vi "thcd401_get_sp_value.vi"(7 "channel":u8=1 min=1 max=4 step=1, 8 "error in":errorcluster, 11 "conn_id_in":refnum<k5>) -> (0 "error out":errorcluster, 1 "value":dbl, 2 "value_array":dbl[](array[numeric]), 3 "conn_id_out":refnum<k5>, 4 "status":bool)   [LabVIEW 2019]
panel:
  out "channel_array":i8[](array[numeric])
  out "data_array":string[](array[string])
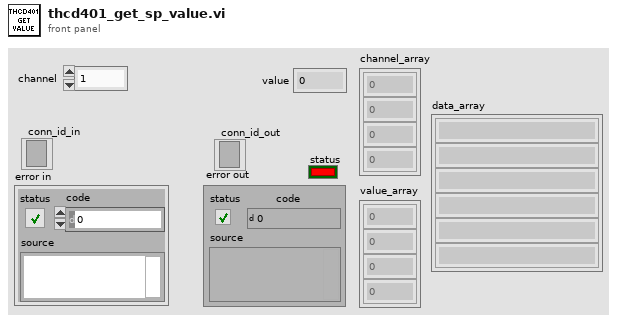
[diagram p1: front panel]
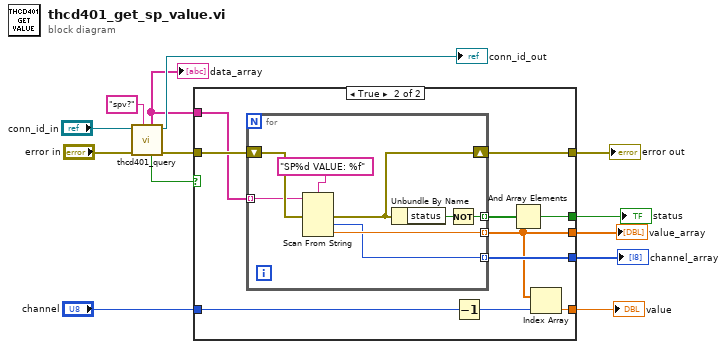
[diagram p0: block diagram]
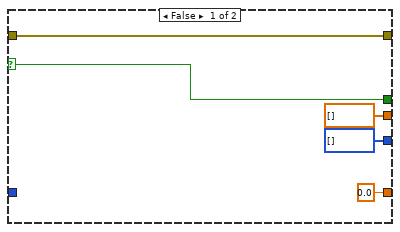
[diagram p2: hidden frame]
diagram:
  n1 = call "thcd401_query.vi"("command"="spv?" ("string"), "error in"="error in", "conn_id_in"="conn_id_in") -> ("error out"=w8:errorcluster, "conn_id_out"=→"conn_id_out":refnum<k5>, "status"=w6:bool, "data_array"=w9:string[])  [unwired: 5 in]
  "data_array" <- w9
  n2 = case shown="True" w6 {
    selector: w6 -> [w17 _]
    tunnel: w9 -> [_ w24]
    tunnel: w8 -> [w18 w28]
    tunnel: [dbl[] [] w22] -> w4
    tunnel: [w18 w27] -> w7
    tunnel: [w17 w26] -> w5
    tunnel: [i32[] [] w23] -> w3
    tunnel: [0.0 w20] -> w2
    tunnel: "channel" -> [_ w19]
    frame False {
    }
    frame True {
      n3 = for {
        tunnel: [w32] -> w25 mode=indexing
        shift-right: [w34] -> w27
        shift-left: w28 -> [w36]
        tunnel: [w31] -> w22 mode=indexing
        tunnel: [w30] -> w23 mode=indexing
        tunnel: w24 -> [w29] mode=indexing
        n4 = Scan From String(format string="SP%d VALUE: %f", input string=w29, error in=w36) -> (error out=w34:errorcluster, output 1=w30:i32, output 2=w31:dbl)  [unwired: 3 in, 2 out]
        n5 = Unbundle By Name(w34) -> ("status"=w33:bool)
        n6 = Not(x=w33) -> (.not. x?=w32:bool)
      }
      n7 = Decrement(x=w19) -> (x-1=w21:u8)
      n8 = And Array Elements(Boolean array=w25) -> (logical AND=w26:bool)
      n9 = Index Array(array=w22, index=w21) -> (element=w20:dbl)
    }
  }
  "error out" <- w7
  "status" <- w5
  "value_array" <- w4
  "value" <- w2
  "channel_array" <- w3
